vi "Calibration Helper2.vi"(7 "Std Devs":cluster{"H":dbl, "S":dbl, "V":dbl}={"H"=4.0, "S"=6.0, "V"=6.0}, 8 "Color Mode":u16(ring)=2 items=["RGB", "HSL", "HSV", "HSI", "CIE L*a*b*", "CIE XYZ"], 9 "Color Components":T1={"Hue"={110.0, 142.0}, "Sat"={138.0, 255.0}, "Val"={139.0, 198.0}} {"Val" scale=0.0..255.0; "Sat" scale=0.0..255.0; "Hue" scale=0.0..255.0 scale format="%#_3g"}, 10 "Image":T2, 11 "Image Ctl Refnum":refnum<vi>) -> (2 "Changed":bool, 3 "output color":T3)   [LabVIEW 2015]
doc: "Use the ROI (region of interest) to mask the image and compute a histogram of the indicated region. This provides the average H, S, and V values as well as the\nstandard deviation of each. It then calculates the initial upper and lower values we want to use for the threshold, and ensure that they are between 0 and 255. Hue, or the 0'th item is\na circular coordinate, so we sometimes flip the upper and lower when the computed value wraps past zero. The other values are linear and are simply clamped. This statistical approach is a reasonable approach when the ROI makes sense, but it is often useful to adjust the high/low values after the auto-calibration."
uses:
  <vilib>/vision/Image Controls.llb/IMAQ Image.ctl
  <vilib>/vision/NI_Vision_Development_Module.lvlib
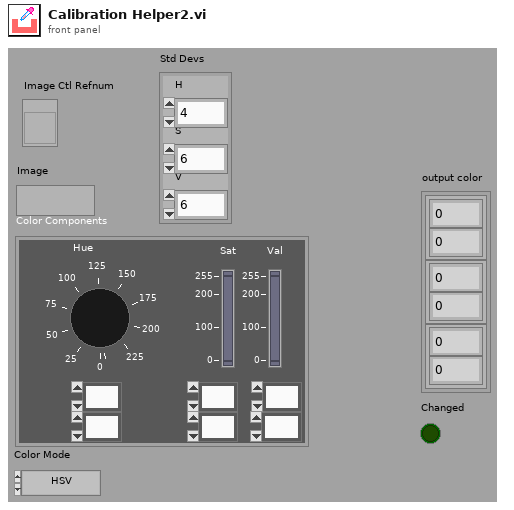
[diagram p1: front panel]
types:
  T1 = cluster{"Hue":cluster{dbl, dbl}, "Sat":cluster{dbl, dbl}, "Val":cluster{dbl, dbl}}
  T2 = typedef "IMAQ Image.ctl" = refnum<image>
  T3 = cluster{cluster{dbl, dbl}, cluster{dbl, dbl}, cluster{dbl, dbl}}
  T4 = typedef "Image Type" = u32
  T5 = cluster{"Global Rectangle":i32[], "Contours":cluster{"Contour Type":u32, "ROI Type":u32, "Points":i32[]}[]}
  T6 = cluster{"histogram":u32[], "Minimal Value":sgl, "Maximal Value":sgl, "Starting Value":sgl, "Interval Width":sgl, "Mean Value":sgl, "Standard  Variation":sgl, "Area (pixels)":i32}
  T7 = cluster{"histogram":u32[], "Minimal Value":sgl, "Maximal Value":sgl, "Starting Value":sgl, "Interval Width":sgl, "Mean Value":sgl, "Standard  Variation":sgl, "Area (pixels)":i32}[]
  T8 = cluster{"[0]":cluster{dbl, dbl}, "[1]":cluster{dbl, dbl}, "[2]":cluster{dbl, dbl}}
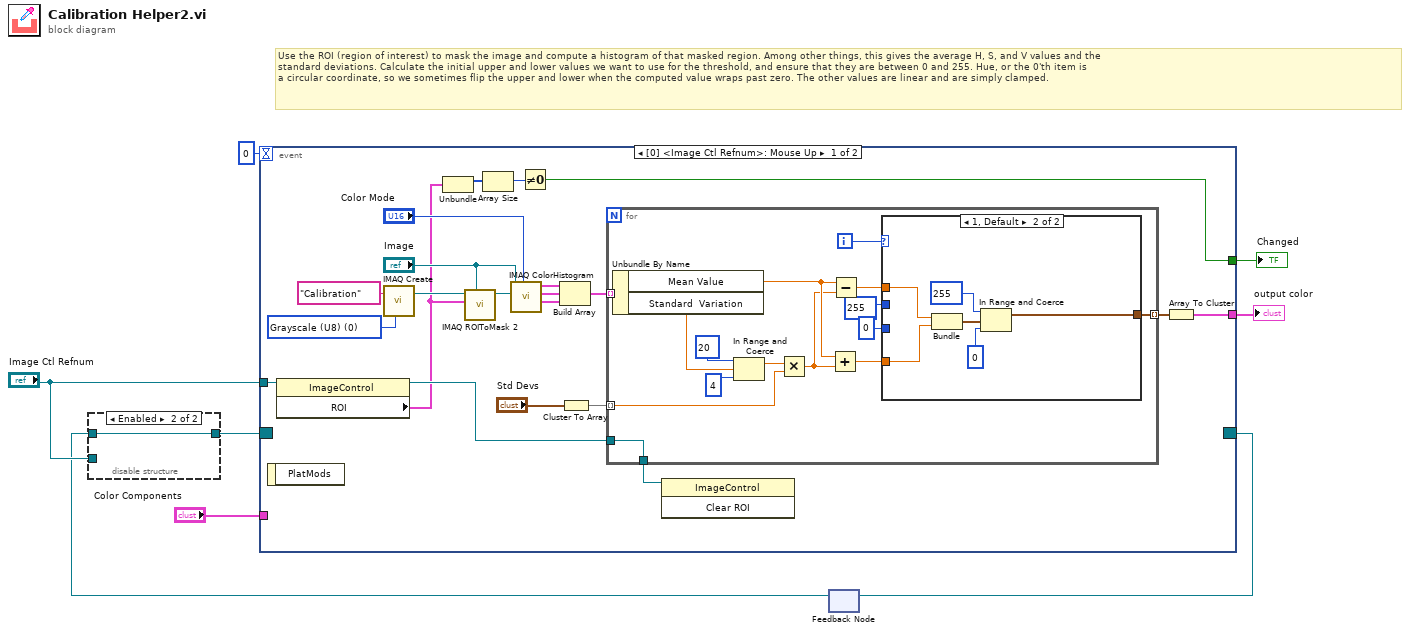
[diagram p0: block diagram]
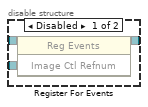
[diagram p2: hidden frame]
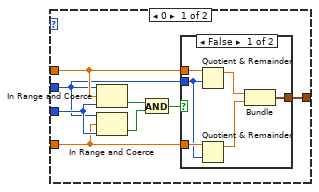
[diagram p3: hidden frame]
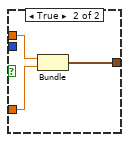
[diagram p4: hidden frame]
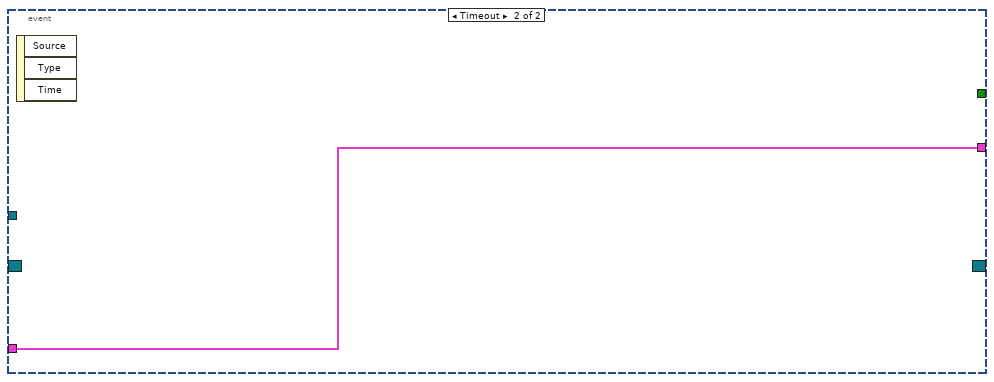
[diagram p5: hidden frame]
diagram:
  # "Use the ROI (region of interest) to mask the image and compute a histogram of that masked region. Among other things, this gives the average H, S, and V values and the\nstandard deviations. Calculate the initial upper and lower values we want to use for the threshold, and ensure that they are between 0 and 255. Hue, or the 0'th item is\na circular coordinate, so we sometimes flip the upper and lower when the computed value wraps past zero. The other values are linear and are simply clamped."
  n1 = feedback #1() -> (w2:refnum<event-registration>)  [unwired: 1 in]
  n2 = disable-structure shown="Enabled" {
    disable-tunnel: "Image Ctl Refnum" -> [w11 _]
    disable-tunnel: [w10 w12] -> w6
    disable-tunnel: w2 -> [w9 w12]
    frame Disabled {
      n3 = register-events(reference=w9, w11) -> (reference out=w10:refnum<event-registration>)  [unwired: 1 in, 1 out]
    }
    frame Enabled {
    }
  }
  n4 = event shown="[0] <Image Ctl Refnum>: Mouse Up" {
    selector: w6 -> [_ _]
    dyn-events: [_ _] -> w3
    timeout: 0 -> [_ _]
    tunnel: "Image Ctl Refnum" -> [w20 _]
    tunnel: "Color Components" -> [_ w72]
    tunnel: [w17 w72] -> w4
    tunnel: [w13 _] -> w1
    event Mouse Up {
      w33 = T4 0 items=["Grayscale (U8)", "Grayscale (I16)", "Grayscale (SGL)", "Complex (CSG)", "RGB (U32)", "HSL (U32)", "RGB (U64)", "Grayscale (U16)"] ("Image Type")
      n5 = event-data() -> ()  [unwired: 1 in, 1 out]
      n6 = property on="Property Node" class="ImageControl"(reference=w20) -> (reference out=w18:refnum<vi>, "ROI"=w16:T5)  [unwired: 1 in, 1 out]
      n7 = call "IMAQ Create"("Image Name"="Calibration", "Image Type"=w33) -> ("New Image"=w30:T2)  [unwired: 3 in, 1 out]
      n8 = Unbundle(w16) -> ("Global Rectangle"=w15:i32[])  [unwired: 1 out]
      n9 = call "IMAQ ROIToMask 2"("Image Model"="Image", "ROI Descriptor"=w16, "Image"=w30) -> ("Image Out"=w31:T2)  [unwired: 6 in, 2 out]
      n10 = Array Size(array=w15) -> (size(s)=w14:i32)
      n11 = call "IMAQ ColorHistogram"("Color Mode"="Color Mode", "Image Src"="Image", "Image Mask"=w31) -> ("Red or Hue or X or L* Histogram Report"=w26:T6, "Green or Sat or Y or a* Histogram Report"=w25:T6, "Blue or Luma or Val or Inten or Z or b* Histogram Report"=w24:T6)  [unwired: 3 in, 1 out]
      n12 = Not Equal To 0?(x=w14) -> (x != 0?=w13:bool)
      n13 = Build Array(w26, w25, w24) -> (w22:T7)
      n14 = Cluster To Array(cluster="Std Devs") -> (array=w23:dbl[])
      n15 = for {
        tunnel: w23 -> [w44] mode=indexing
        tunnel: w22 -> [w48] mode=indexing
        tunnel: [w39] -> w21 mode=indexing
        tunnel: [w34] -> w19
        tunnel: w18 -> [w34]
        i -> [w37]
        n16 = Unbundle By Name(w48) -> ("Mean Value"=w42:sgl, "Standard  Variation"=w45:sgl)
        n17 = In Range and Coerce(upper limit=20, x=w45, lower limit=4) -> (coerced(x)=w43:sgl)  [unwired: 1 out]
        n18 = Multiply(x=w43, y=w44) -> (x*y=w38:dbl)
        n19 = Add(x=w42, y=w38) -> (x+y=w40:dbl)
        n20 = Subtract(x=w42, y=w38) -> (x-y=w41:dbl)
        n21 = case shown="1, Default" w37 {
          tunnel: w41 -> [w51 w68]
          tunnel: w40 -> [w50 w67]
          tunnel: [w53 w66] -> w39
          tunnel: 255 -> [w49 _]
          tunnel: 0 -> [w52 _]
          frame 0 {
            n22 = In Range and Coerce(upper limit=w49, x=w51, lower limit=w52) -> (In Range?=w55:bool)  [unwired: 1 out]
            n23 = In Range and Coerce(upper limit=w49, x=w50, lower limit=w52) -> (In Range?=w54:bool)  [unwired: 1 out]
            n24 = And(x=w55, y=w54) -> (x .and. y?=w56:bool)
            n25 = case shown="False" w56 {
              tunnel: [w59 w65] -> w53
              tunnel: w51 -> [w62 w63]
              tunnel: w50 -> [w61 w64]
              tunnel: w49 -> [w60 _]
              frame False {
                n26 = Quotient & Remainder(x=w62, y=w60) -> (x-y*floor(x/y)=w57:dbl)  [unwired: 1 out]
                n27 = Quotient & Remainder(x=w61, y=w60) -> (x-y*floor(x/y)=w58:dbl)  [unwired: 1 out]
                n28 = Bundle(w57, w58) -> (w59:cluster{dbl, dbl})  [unwired: 1 in]
              }
              frame True {
                n29 = Bundle(w63, w64) -> (w65:cluster{dbl, dbl})  [unwired: 1 in]
              }
            }
          }
          frame 1, Default {
            n30 = Bundle(w68, w67) -> (w71:cluster{dbl, dbl})  [unwired: 1 in]
            n31 = In Range and Coerce(upper limit=255, x=w71, lower limit=0) -> (coerced(x)=w66:cluster{dbl, dbl})  [unwired: 1 out]
          }
        }
      }
      n32 = invoke on="Invoke Node" class="ImageControl" method="Clear ROI"(reference=w19) -> ()  [unwired: 2 in, 3 out]
      n33 = Array To Cluster(array=w21) -> (cluster=w17:T8)
    }
    event Timeout {
      n34 = event-data() -> ()  [unwired: 1 in, 3 out]
    }
  }
  "output color" <- w4
  "Changed" <- w1
  n35 = feedback-in #1(w3) -> ()
